vi "new.vi"(7 "ID":string, 9 "task token":refnum<class "null task token.lvclass">, 10 "results reporter":refnum<class "results reporter.lvclass">, 11 "timer":i32) -> (3 "noncancellable wait out":refnum<class "noncancellable wait.lvclass">)   [LabVIEW 2013, in "noncancellable wait.lvclass"]
uses:
  noncancellable wait.lvclass
  task token/null task token.lvclass
  results reporter/results reporter.lvclass
  noncancellable wait.lvclass/noncancellable wait.ctl
  task/task.lvclass
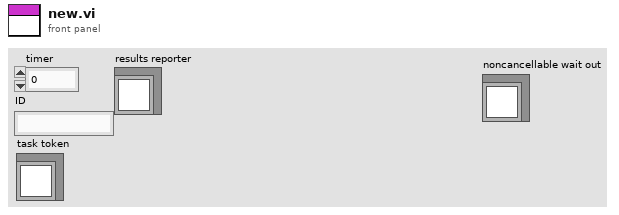
[diagram p1: front panel]
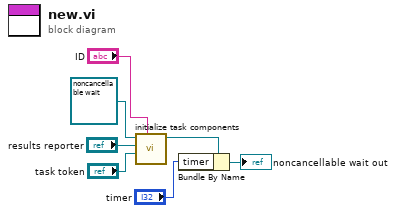
[diagram p0: block diagram]
diagram:
  n1 = call "initialize task components.vi"("ID"="ID", "task token"="task token", "results reporter"="results reporter", "task in"=refnum<class "noncancellable wait.lvclass"> refnum ("noncancellable wait in")) -> ("task out"=w6:refnum<class "noncancellable wait.lvclass">)  [unwired: 7 in]
  n2 = Bundle By Name(cluster=w6, "timer"="timer") -> (→"noncancellable wait out":refnum<class "noncancellable wait.lvclass">)
